vi "IP Address.vi"() -> ()   [LabVIEW 2017]
panel:
  in  "IP Address":string="169.254.150.69:6969"
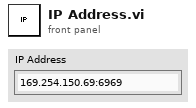
[diagram p1: front panel]
diagram:
